vi "ProcessCalibrationInputs.vi"(10 "Point":i32[](array[numeric]), 11 "ExperimentVariables":T1={"Calibration Input"=[], "CalibrationResults"={"Center in Pixels"=[374.0120339529387, 375.46592887074246], "Angle"=0.022945275255000355, "Pixels/MHz X"=0.0, "Pixels/MHz Y"=0.0}, "Highlight"=[], "Running Script"=refnum}) -> (1 "Status":enum16{"Finished", "Waiting"}(ring), 3 "output cluster":T1={"Calibration Input"=[], "CalibrationResults"={"Center in Pixels"=[374.0120339529387, 375.46592887074246], "Angle"=0.022945275255000355, "Pixels/MHz X"=0.0, "Pixels/MHz Y"=0.0}, "Highlight"=[], "Running Script"=refnum})   [LabVIEW 2017]
uses:
  ExperimentVariables.ctl
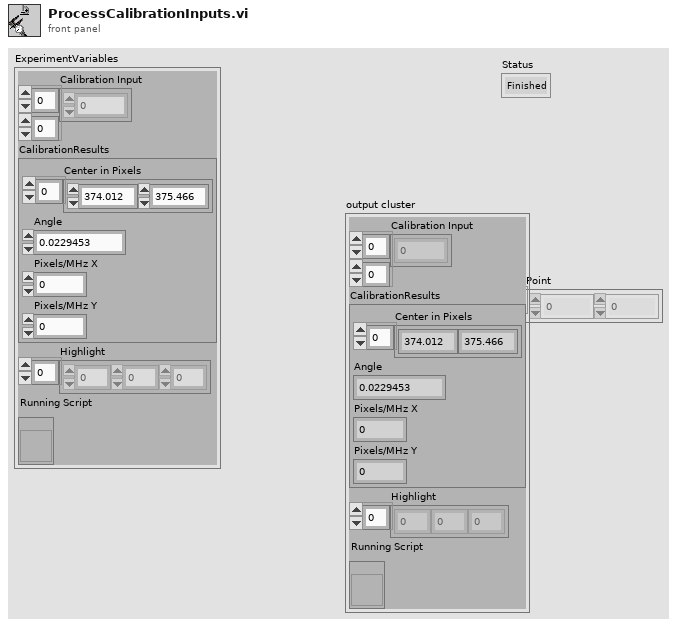
[diagram p1: front panel]
types:
  T1 = typedef "ExperimentVariables.ctl" = cluster{"Calibration Input":i32[][], "CalibrationResults":cluster{"Center in Pixels":dbl[], "Angle":dbl, "Pixels/MHz X":dbl, "Pixels/MHz Y":dbl}, "Highlight":i32[], "Running Script":refnum<vi>}
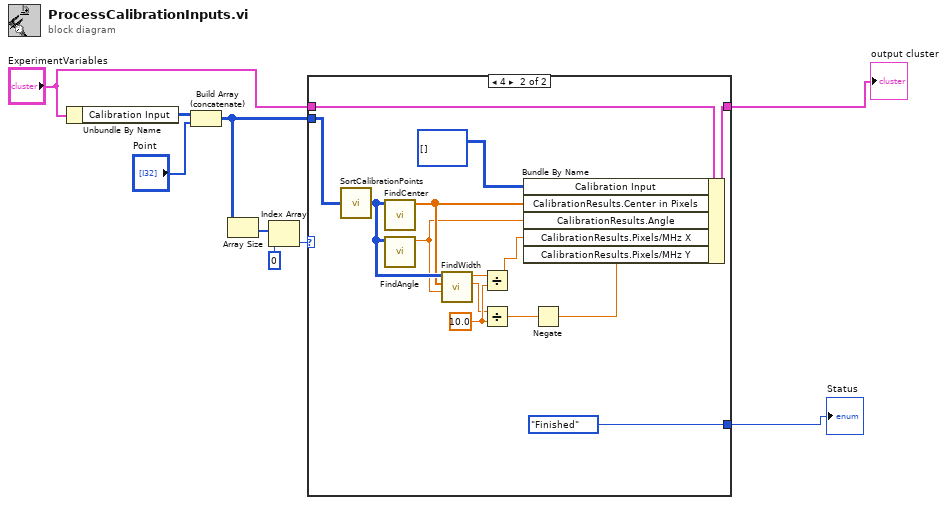
[diagram p0: block diagram]
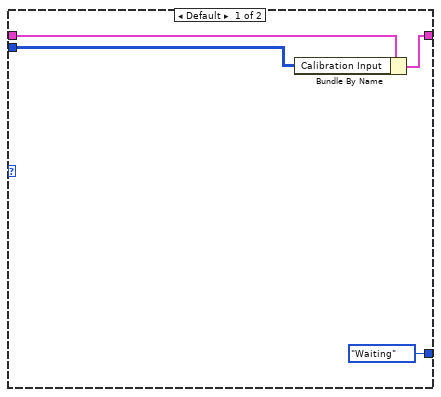
[diagram p2: hidden frame]
diagram:
  n1 = Unbundle By Name("ExperimentVariables") -> ("Calibration Input"=w5:i32[][])
  n2 = Build Array (concatenate)(w5, "Point") -> (w4:i32[][])
  n3 = Array Size(array=w4) -> (size(s)=w7:i32[])
  n4 = Index Array(array=w7, index=0) -> (element=w9:i32)
  n5 = case shown="4" w9 {
    tunnel: w4 -> [w11 w26]
    tunnel: "ExperimentVariables" -> [w13 w25]
    tunnel: [w12 w22] -> w2
    tunnel: [enum16{"Finished", "Waiting"}."Waiting" ("Status") enum16{"Finished", "Waiting"}."Finished" ("Status")] -> w1
    frame Default {
      n6 = Bundle By Name(cluster=w13, "Calibration Input"=w11) -> (w12:T1)
    }
    frame 4 {
      w20 = 10.0 ("y")
      n7 = call "SortCalibrationPoints.vi"("Array in"=w26) -> ("Array out"=w27:i32[][])
      n8 = call "FindCenter.vi"("Array in"=w27) -> ("Center"=w24:dbl[])  [unwired: 10 in]
      n9 = call "FindAngle.vi"("Array in"=w27) -> ("Angle"=w23:dbl)  [unwired: 10 in]
      n10 = call "FindWidth.vi"("theta"=w23, "Center"=w24, "Array in"=w27) -> ("height"=w19:dbl, "width"=w18:dbl)  [unwired: 4 in]
      n11 = Divide(x=w18, y=w20) -> (x/y=w14:dbl)
      n12 = Divide(x=w19, y=w20) -> (x/y=w16:dbl)
      n13 = Negate(x=w16) -> (-x=w15:dbl)
      n14 = Bundle By Name(cluster=w25, "Calibration Input"=i32[][] [], "CalibrationResults.Center in Pixels"=w24, "CalibrationResults.Angle"=w23, "CalibrationResults.Pixels/MHz X"=w14, "CalibrationResults.Pixels/MHz Y"=w15) -> (w22:T1)
    }
  }
  "output cluster" <- w2
  "Status" <- w1
